vi "Samples.vi"() -> ()   [LabVIEW 2012]
panel:
  in  "Samples":T1
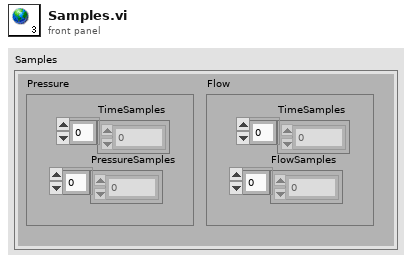
[diagram p1: front panel]
types:
  T1 = cluster{"Pressure":cluster{"TimeSamples":dbl[], "PressureSamples":dbl[]}, "Flow":cluster{"TimeSamples":dbl[], "FlowSamples":dbl[]}}
diagram:
